vi "Output Audio.vi"(8 "error in (no error)":errorcluster, 10 "Instrument In":variant) -> (0 "error out":errorcluster, 2 "Instrument out":variant)   [LabVIEW 2014, in "mySynthesizer.lvlib"]
uses:
  mySynthesizer.lvlib
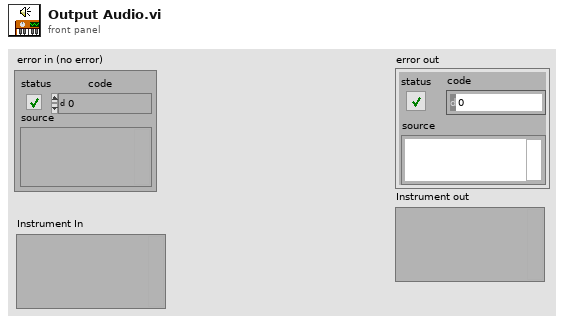
[diagram p1: front panel]
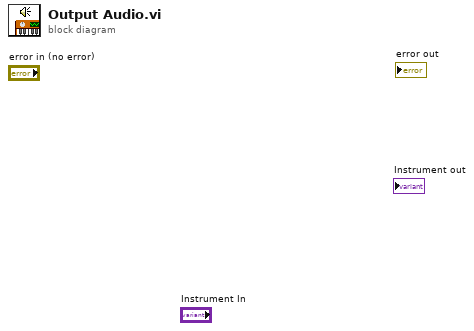
[diagram p0: block diagram]
diagram:
